vi "apply page settings.vi"(8 "error in (no error)":errorcluster, 10 "page settings":string, 11 "tab control refnum":refnum<vi>) -> (0 "error out":errorcluster)   [LabVIEW 2024, in "controls manager.lvlib"]
uses:
  controls manager.lvlib
  <vilib>/Utility/error.llb/Trim Whitespace One-Sided.vi
  <vilib>/Utility/error.llb/Error Cluster From Error Code.vi
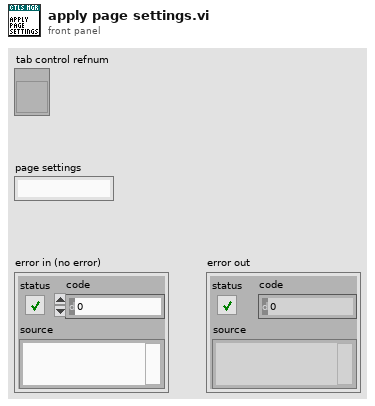
[diagram p1: front panel]
types:
  T1 = enum32{"Page Enabled", "Page Disabled", "Page Disabled & Grayed"}
  T2 = typedef "controls manager.lvlib/keywords.ctl" = enum16{"___", "enable", "disable", "gray", "visible", "hidden", "tip", "caption", "blinking", "not_blinking", "page", "default"}
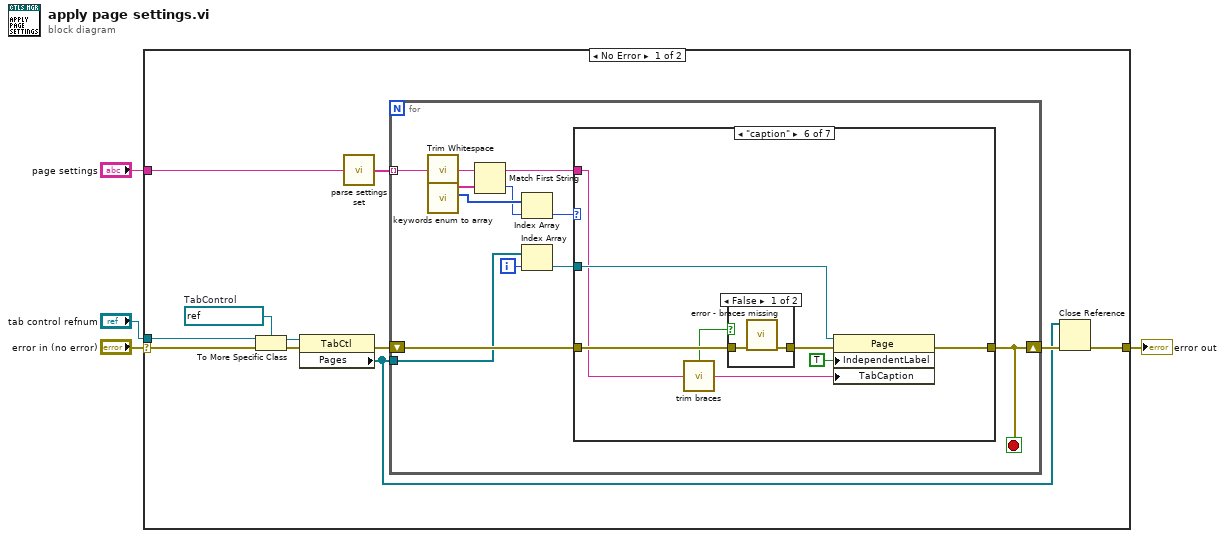
[diagram p0: block diagram]
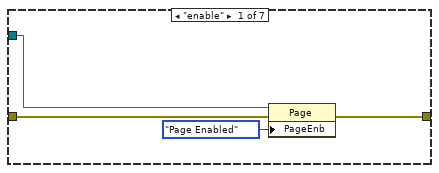
[diagram p2: hidden frame]
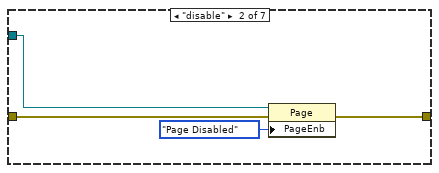
[diagram p3: hidden frame]
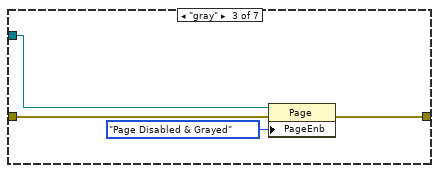
[diagram p4: hidden frame]
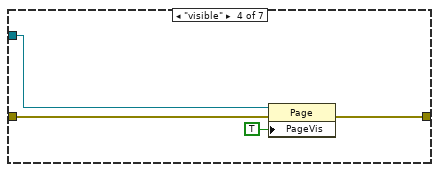
[diagram p5: hidden frame]
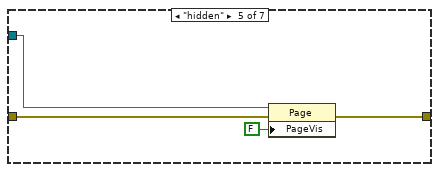
[diagram p6: hidden frame]
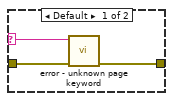
[diagram p9: hidden frame]
diagram:
  n1 = case shown="No Error" "error in (no error)" {
    selector: "error in (no error)" -> [w13 w66]
    tunnel: "tab control refnum" -> [w15 _]
    tunnel: "page settings" -> [w14 _]
    tunnel: [w6 w66] -> w1
    frame No Error {
      w11 = refnum<vi> refnum  # TabControl
      n2 = To More Specific Class(target class=w11, reference=w15, error in=w13) -> (specific class reference=w8:refnum<vi>, error out=w10:errorcluster)
      n3 = property class="TabCtl"(reference=w8, error in=w10) -> (error out=w9:errorcluster, "Pages"=w5:refnum<vi>[])  [unwired: 1 out]
      n4 = call "parse settings set.vi"("settings in"=w14) -> ("settings out"=w7:string[])
      n5 = for {
        tunnel: w5 -> [w20]
        tunnel: w7 -> [w21] mode=indexing
        shift-right: [w16] -> w12
        shift-left: w9 -> [w22]
        i -> [w19]
        stop <- w16 stop-if-true
        n6 = call <vilib>:"Trim Whitespace.vi"("string"=w21) -> ("trimmed string"=w17:string)  [unwired: 1 in]
        n7 = call "keywords enum to array.vi"() -> ("enums"=w26:T2[], "strings"=w25:string[])  [unwired: 10 in]
        n8 = Match First String(2:w25, 3:w17) -> (0:w24:i32, 1:w23:string)
        n9 = Index Array(array=w26, index=w24) -> (element=w27:T2)
        n10 = Index Array(array=w20, index=w19) -> (element=w18:refnum<vi>)
        n11 = case shown="\"caption\"" w27 {
          tunnel: w23 -> [_ _ _ _ _ w51 w59]
          tunnel: w22 -> [w31 w35 w39 w43 w47 w55 w61]
          tunnel: [w30 w34 w38 w42 w46 w54 w60] -> w16
          tunnel: w18 -> [w29 w33 w37 w41 w45 w53 _]
          frame "enable" {
            n12 = property class="Page"(reference=w29, error in=w31, "PageEnb"=T1."Page Enabled") -> (error out=w30:errorcluster)  [unwired: 1 out]
          }
          frame "disable" {
            n13 = property class="Page"(reference=w33, error in=w35, "PageEnb"=T1."Page Disabled") -> (error out=w34:errorcluster)  [unwired: 1 out]
          }
          frame "gray" {
            n14 = property class="Page"(reference=w37, error in=w39, "PageEnb"=T1."Page Disabled & Grayed") -> (error out=w38:errorcluster)  [unwired: 1 out]
          }
          frame "visible" {
            n15 = property class="Page"(reference=w41, error in=w43, "PageVis"=TRUE ("Page Visible")) -> (error out=w42:errorcluster)  [unwired: 1 out]
          }
          frame "hidden" {
            n16 = property class="Page"(reference=w45, error in=w47, "PageVis"=FALSE ("Page Visible")) -> (error out=w46:errorcluster)  [unwired: 1 out]
          }
          frame "caption" {
            n17 = call "trim braces.vi"("string"=w51) -> ("braces?"=w48:bool, "trimmed string"=w50:string)
            n18 = case shown="False" w48 {
              tunnel: w55 -> [w57 w58]
              tunnel: [w56 w58] -> w49
              frame False {
                n19 = call "error - braces missing.vi"("error in (no error)"=w57) -> ("error out"=w56:errorcluster)  [unwired: 10 in]
              }
              frame True {
              }
            }
            n20 = property class="Page"(reference=w53, error in=w49, "IndependentLabel"=TRUE, "TabCaption"=w50) -> (error out=w54:errorcluster)  [unwired: 1 out]
          }
          frame Default {
            n21 = case shown="\"\", \"nothing\", \"null\"" w59 {
              selector: w59 -> [w62 _]
              tunnel: w61 -> [w64 w65]
              tunnel: [w63 w65] -> w60
              frame Default {
                n22 = call "error - unknown page keyword.vi"("error in (no error)"=w64, "keyword"=w62) -> ("error out"=w63:errorcluster)  [unwired: 9 in]
              }
              frame "", "nothing", "null" {
              }
            }
          }
        }
      }
      n23 = Close Reference(reference=w5, error in (no error)=w12) -> (error out=w6:errorcluster)
    }
    frame Error {
    }
  }
  "error out" <- w1
